vi "Decode Output.vi"(10 "Map of numbers":T1[](array[typedef]), 11 "array type (2D Dbl)":string[](array[string])) -> (2 "Numeric":i32, 3 "String":string)   [LabVIEW 2019, in "Day 8.lvlib"]
uses:
  Day 8.lvlib
  Controls/Digit.ctl
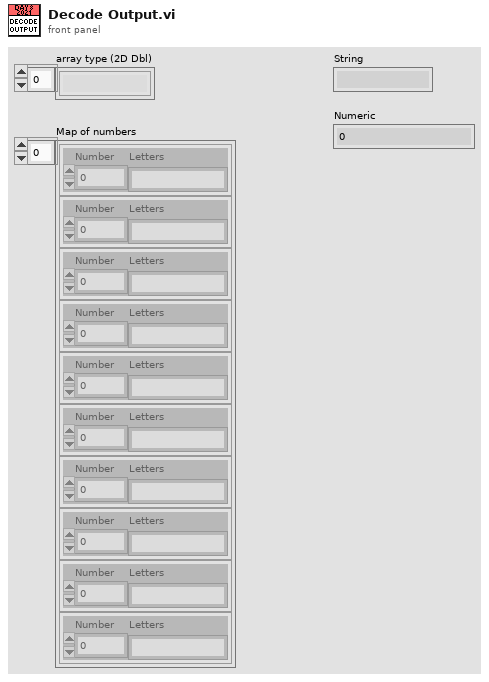
[diagram p1: front panel]
types:
  T1 = typedef "Day 8.lvlib/Digit.ctl" = cluster{"Number":u8, "Letters":string}
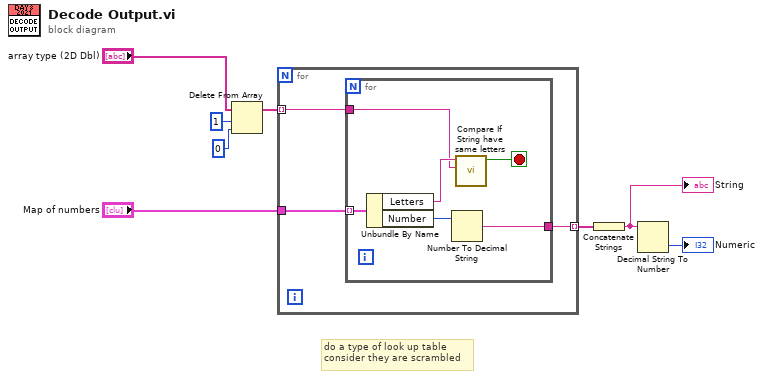
[diagram p0: block diagram]
diagram:
  # "do a type of look up table\nconsider they are scrambled"
  n1 = Delete From Array(array="array type (2D Dbl)", length=1, index=0) -> (array with subset deleted=w6:string[])  [unwired: 1 out]
  n2 = for {
    tunnel: w6 -> [w11] mode=indexing
    tunnel: "Map of numbers" -> [w10]
    tunnel: [w9] -> w1 mode=indexing
    n3 = for {
      tunnel: w11 -> [w15]
      tunnel: w10 -> [w17] mode=indexing
      tunnel: [w13] -> w9
      stop <- w12 stop-if-true
      n4 = Unbundle By Name(w17) -> ("Letters"=w16:string, "Number"=w14:u8)
      n5 = Number To Decimal String(number=w14) -> (decimal integer string=w13:string)  [unwired: 1 in]
      n6 = call "Compare If String have same letters.vi"("format string"=w15, "Letters"=w16) -> ("Same Letters?"=w12:bool)  [unwired: 9 in]
    }
  }
  n7 = Concatenate Strings(w1) -> (w8:string)
  "String" <- w8
  n8 = Decimal String To Number(string=w8) -> (number=→"Numeric":i32)  [unwired: 2 in, 1 out]
